vi "Clean Timestamp.vi"(11 "Time Stamp":timestamp) -> (3 "Clean time stamp":timestamp)   [LabVIEW 2012]
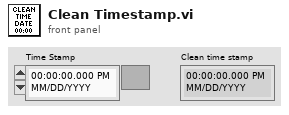
[diagram p1: front panel]
types:
  T1 = typedef "LVDateTimeRec.ctl" = cluster{"fractional second":dbl, "second":i32, "minute":i32, "hour":i32, "day of month":i32, "month":i32, "year":i32, "day of week":i32, "day of year":i32, "DST":i32}
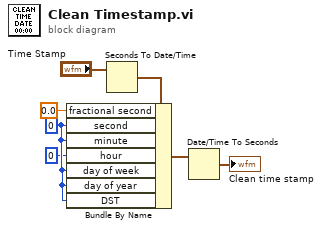
[diagram p0: block diagram]
diagram:
  w5 = 0 ("second")
  n1 = Seconds To Date/Time(time stamp (now)="Time Stamp") -> (date time rec=w3:T1)  [unwired: 1 in]
  n2 = Bundle By Name(cluster=w3, "fractional second"=0.0, "second"=w5, "minute"=w5, "hour"=0, "day of week"=w5, "day of year"=w5, "DST"=w5) -> (w6:T1)
  n3 = Date/Time To Seconds(2:w6) -> (0:→"Clean time stamp":timestamp)  [unwired: 1 in]
